vi "NewEnchantedRoom.vi"(8 "error in (no error)":errorcluster, 10 "Spell":refnum<class "Spell.lvclass">, 11 "RoomNumber":i32) -> (0 "error out":errorcluster, 3 "EnchantedRoom":refnum<class "EnchantedRoom.lvclass">)   [LabVIEW 2020, in "EnchantedRoom.lvclass"]
uses:
  EnchantedRoom.lvclass
  Spell/Spell.lvclass
  Support/Class/ConsoleOutput.lvclass
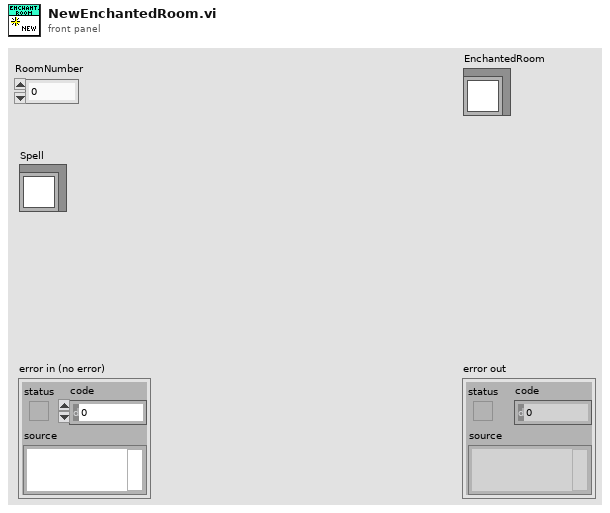
[diagram p1: front panel]
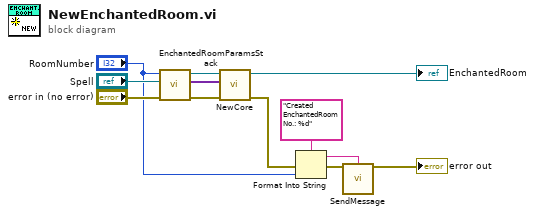
[diagram p0: block diagram]
diagram:
  n1 = call "EnchantedRoomParamsStack.vi"("error in (no error)"="error in (no error)", "Spell"="Spell", "RoomNumber"="RoomNumber") -> ("error out"=w12:errorcluster, "HierarchyParams"=w11:variant[], "EnchantedRoom"=w10:refnum<class "EnchantedRoom.lvclass">)  [unwired: 6 in]
  n2 = call-dynamic "NewCore.vi"("error in (no error)"=w12, "ParamsArray"=w11, "EnchantedRoom"=w10) -> ("error out"=w3:errorcluster, "EnchantedRoom"=→"EnchantedRoom":refnum<class "EnchantedRoom.lvclass">)  [unwired: 7 in]
  n3 = Format Into String(format string="Created EnchantedRoom No.: %d" ("Message"), error in=w3, "RoomNumber") -> (resulting string=w4:string, error out=w5:errorcluster)  [unwired: 1 in]
  n4 = call "SendMessage.vi"("Message"=w4, "error in (no error)"=w5) -> ("error out"=→"error out":errorcluster)  [unwired: 13 in]
